vi "Set ServerEvent.vi"(8 "error in (no error)":errorcluster, 10 "ServerEvent_Data":T1, 11 "gRPCid":T2) -> (0 "error out":errorcluster, 3 "gRPCid out":T2)   [LabVIEW 2019, in "OOP Server.lvclass"]
uses:
  OOP Server.lvclass
  gRPC interface/Server API/typeDefs/grpcId.ctl
  ServerEvent_Data.ctl
  7bdd4605-c7f7-42bf-87d0-91e104daf0dd.vi
  <vilib>/Utility/error.llb/Error Cluster From Error Code.vi
  gRPC interface/gprc-lvsupport.lvlib
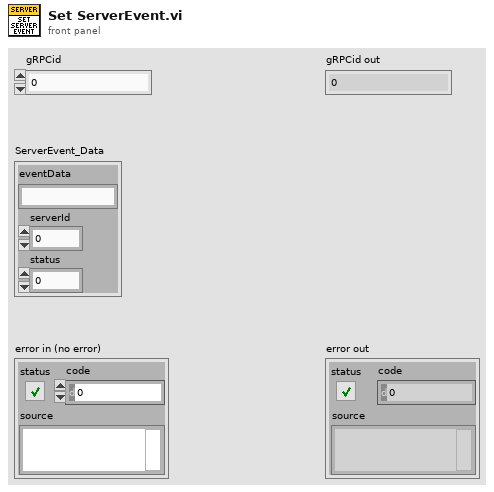
[diagram p1: front panel]
types:
  T1 = typedef "OOP Server.lvclass/ServerEvent_Data.ctl" = cluster{"eventData":string, "serverId":i32, "status":i32}
  T2 = typedef "gprc-lvsupport.lvlib/grpcId.ctl" = u64
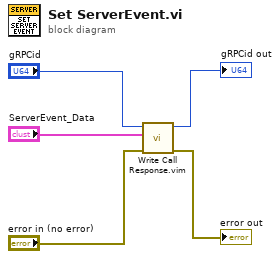
[diagram p0: block diagram]
diagram:
  n1 = call "Write Call Response.vim"("error in (no error)"="error in (no error)", "Response Data"="ServerEvent_Data", "gRPCid in"="gRPCid") -> ("error out"=→"error out":errorcluster, "gRPCid"=→"gRPCid out":T2)  [unwired: 7 in]
